vi "PC Streaming Host with slow.vi"() -> ()   [LabVIEW 2012]
uses:
  <vilib>/userdefined/High Color/nirio_resource_hc.ctl
  <vilib>/FPGAPlugInAG/PXI-7951R/niLvFpga_Open_PXI-7951R.vi
  <vilib>/rvi/interface/common/dynamic/niFpgaDynamicAddResources.vi
  <vilib>/Utility/error.llb/Error Cluster From Error Code.vi
  <vilib>/rvi/errors/niLvFpgaAdjustHostInterfaceError.vi
  <vilib>/FPGAPlugInAG/Dynamic/niLvFpga_Close_Dynamic.vi
  <vilib>/rvi/interface/nirviOpenFPGA/nirviOpenFPGA.xnode
  FPGA Bitfiles/ModuDAQ_FPGATarget_TopLevelFPGAw8ra_+uETqx0Rcow.lvbitx
  <vilib>/rvi/interface/nirviReadWriteControl/nirviReadWriteControl.xnode
  <vilib>/rvi/interface/nirviMethod/nirviMethod.xnode
  <vilib>/rvi/interface/nirviCloseFPGA/nirviCloseFPGA.xnode
  <vilib>/rvi/errors/niLvFpgaMergeErrorWithErrorCode.vi
  <vilib>/ptbypt/NI_PtbyPt.lvlib
  <vilib>/rvi/interface/Simulation/niFpgaSimulationCallBeginRW.vi
  RT_binary.vi
  NiFpgaLv.dll
  <vilib>/FPGAPlugInAG/Dynamic/niLvFpga_ReadFifo_Dynamic.vi
panel:
  out "created path":path
  out "File name":string
  out "Total Data Chunks to Write":dbl
  in  "Tab Control":T1(tab)
  in  "Write mode":bool
  out "directory exists - please wait":u8(slide)
  out "directory ok":bool
  in  "Write Enable":bool
  in  "File Path":path=path "D:/Users/reuterc/Desktop"
  out "File Writing Progress (%)":dbl(slide) scale=0.0..100.0
  in  "Slow Control On":bool
  in  "Fast Data On":bool
  in  "Number of Files to Write":u32=1
  in  "IP Address of NIST Time Server":string(combo)
  in  "VISA resource name":refnum<visa-resource-name>="COM5"
  in  "General Cluster":cluster{"Location":i16} {"Location" items=["Purdue", "NIKHEF", "Zurich", "???"]}
  in  "PXI address":T2 caption="RIO Device"
  in  "Channel Cluster":T3={"det_type"=[], "voltage"=[], "Serial numbers"=[], "Sources"=[], "Trigger level"=[4000, 4000, 4000, 4000, 4000, 4000, 4000, 4000], "Channel On/Off"=[], "Number of Channels"=8}
  in  "Testpulse Cluster":T4={"Master Pulser On/Off"=FALSE, "Testpulse Turnaround Time (samples)"=14, "Pulse Separation (samples)"=0, "Pulse duration (samples)"=0}
  out "Samples per Data Chunk":u32
  in  "DAQ Info Cluster":T5={"Data Chunks per File"=1000, "Samples per Waveform"=95, "Pretrigger Samples"=15, "circular buffer length (samples)"=1000, "Waveforms per Data Chunk"=5000} {"Waveforms per Data Chunk" format="%.2p"}
  out "Average Throughput":dbl(graph)
  out "Loop Time":u32
  out "Inst. Throughput":dbl format="%#_6p"
  out "Elements in FIFO":u32(graph)
  out "FIFO Overflow":bool
  out "Current Chunk":u32
  out "Current File":i32
  out "Waveform Graph":dynamicdata(graph)
  out "Channel number displayed":i16=-1
  in  "Arduino read rate (Hz)":dbl=1.0
  out "read buffer":string
  out "array 2":string[](array[string])
  out "Arduino read failed":bool
  out "Slow time":u64
  out "data":dbl[](array[numeric])
  in  "XON Character":u8=17 format="%.0x"
  in  "XOFF Character":u8=19 format="%.0x"
  out "Slow Cluster":T6={"Number of Slow Parameters"=0, "UTC format?"=TRUE, "Sensor Upper bounds"=[85, 1000000, 8000, 8000, 8000, 14000, 99, 33000], "Sensor Lower bounds"=[-40, 0, -8000, -8000, -8000, -14000, 0, -33000], "datanames"=[], "Descriptions"=[]}
  out "Number of Slow Parameters":i32
  out "FPGA Timestamp (s)":u64
  out "Temperature":dbl(graph)
  out "Pressure":dbl(graph)
  out "magnetic field y coordinate":dbl(graph)
  out "total magnetic field":dbl(graph)
  out "magnetic field z coordinate":dbl(graph)
  out "magnetic field x coordinate":dbl(graph)
  out "humidity":dbl(graph)
  out "XML String":string
  out "error out":errorcluster
  out "NIST Time":u64
  out "NIST Time Failed to Read":bool
  in  "Minutes to wait":u32=5 min=3
  out "UTC format":bool=TRUE
  out "Stopped":bool
  in  "stop 2":bool
  in  "stop":bool
  # "Write continuously"
  # "Write finite number of files"
  # "Program will stop when number of Files to Write is Complete OR if stop is pressed."
  # "TODO: Make this look like the \"detectors\" tab"
  # "Waveform/Data Chunk information"
  # "To compare directly on a scope: Horizontal scale: 200 ns/div Vertical scale: ~100 mV/div If 15 pretriggers, delay = 700 ns"
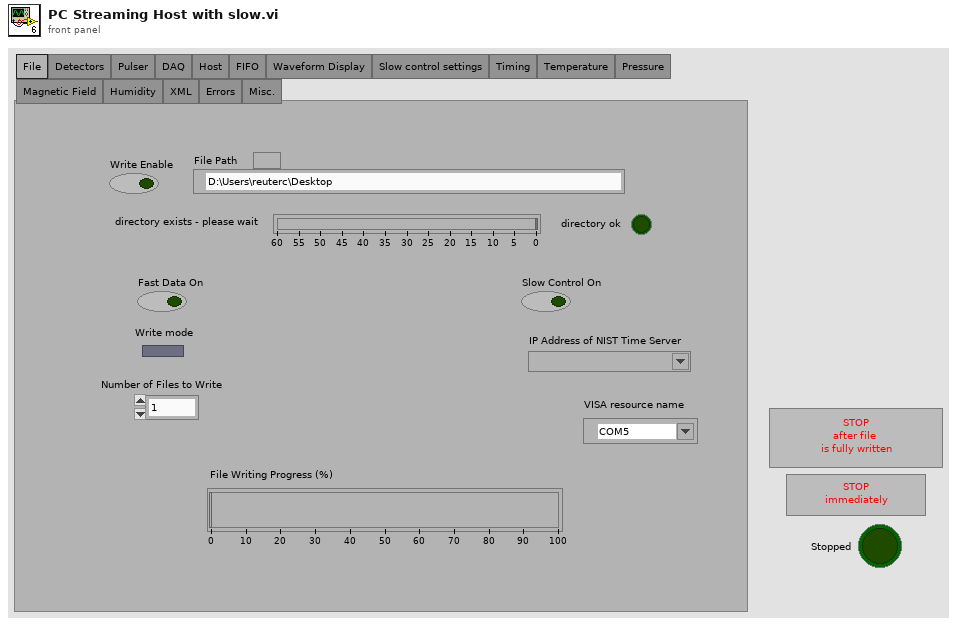
[diagram p1: front panel]
types:
  T1 = enum32{"File", "Detectors", "Pulser", "DAQ", "Host", "FIFO", "Waveform Display", "Slow control settings", "Timing", "Temperature", "Pressure", "Magnetic Field", "Humidity", "XML", "Errors", "Misc."}
  T2 = typedef "nirio_resource_hc.ctl" = tag
  T3 = cluster{"det_type":string[], "voltage":string[], "Serial numbers":string[], "Sources":string[], "Trigger level":i16[], "Channel On/Off":bool[], "Number of Channels":u8}
  T4 = cluster{"Master Pulser On/Off":bool, "Testpulse Turnaround Time (samples)":u32, "Pulse Separation (samples)":u32, "Pulse duration (samples)":u32}
  T5 = cluster{"Data Chunks per File":u32, "Samples per Waveform":u32, "Pretrigger Samples":u32, "circular buffer length (samples)":u32, "Waveforms per Data Chunk":u32}
  T6 = cluster{"Number of Slow Parameters":i32, "UTC format?":bool, "Sensor Upper bounds":i32[], "Sensor Lower bounds":i32[], "datanames":string[], "Descriptions":string[]}
  T7 = enum16{"open", "replace", "create", "open or create", "replace or create", "replace or create with confirmation"}
  T8 = enum16{"big-endian, network order", "native, host order", "little-endian"}
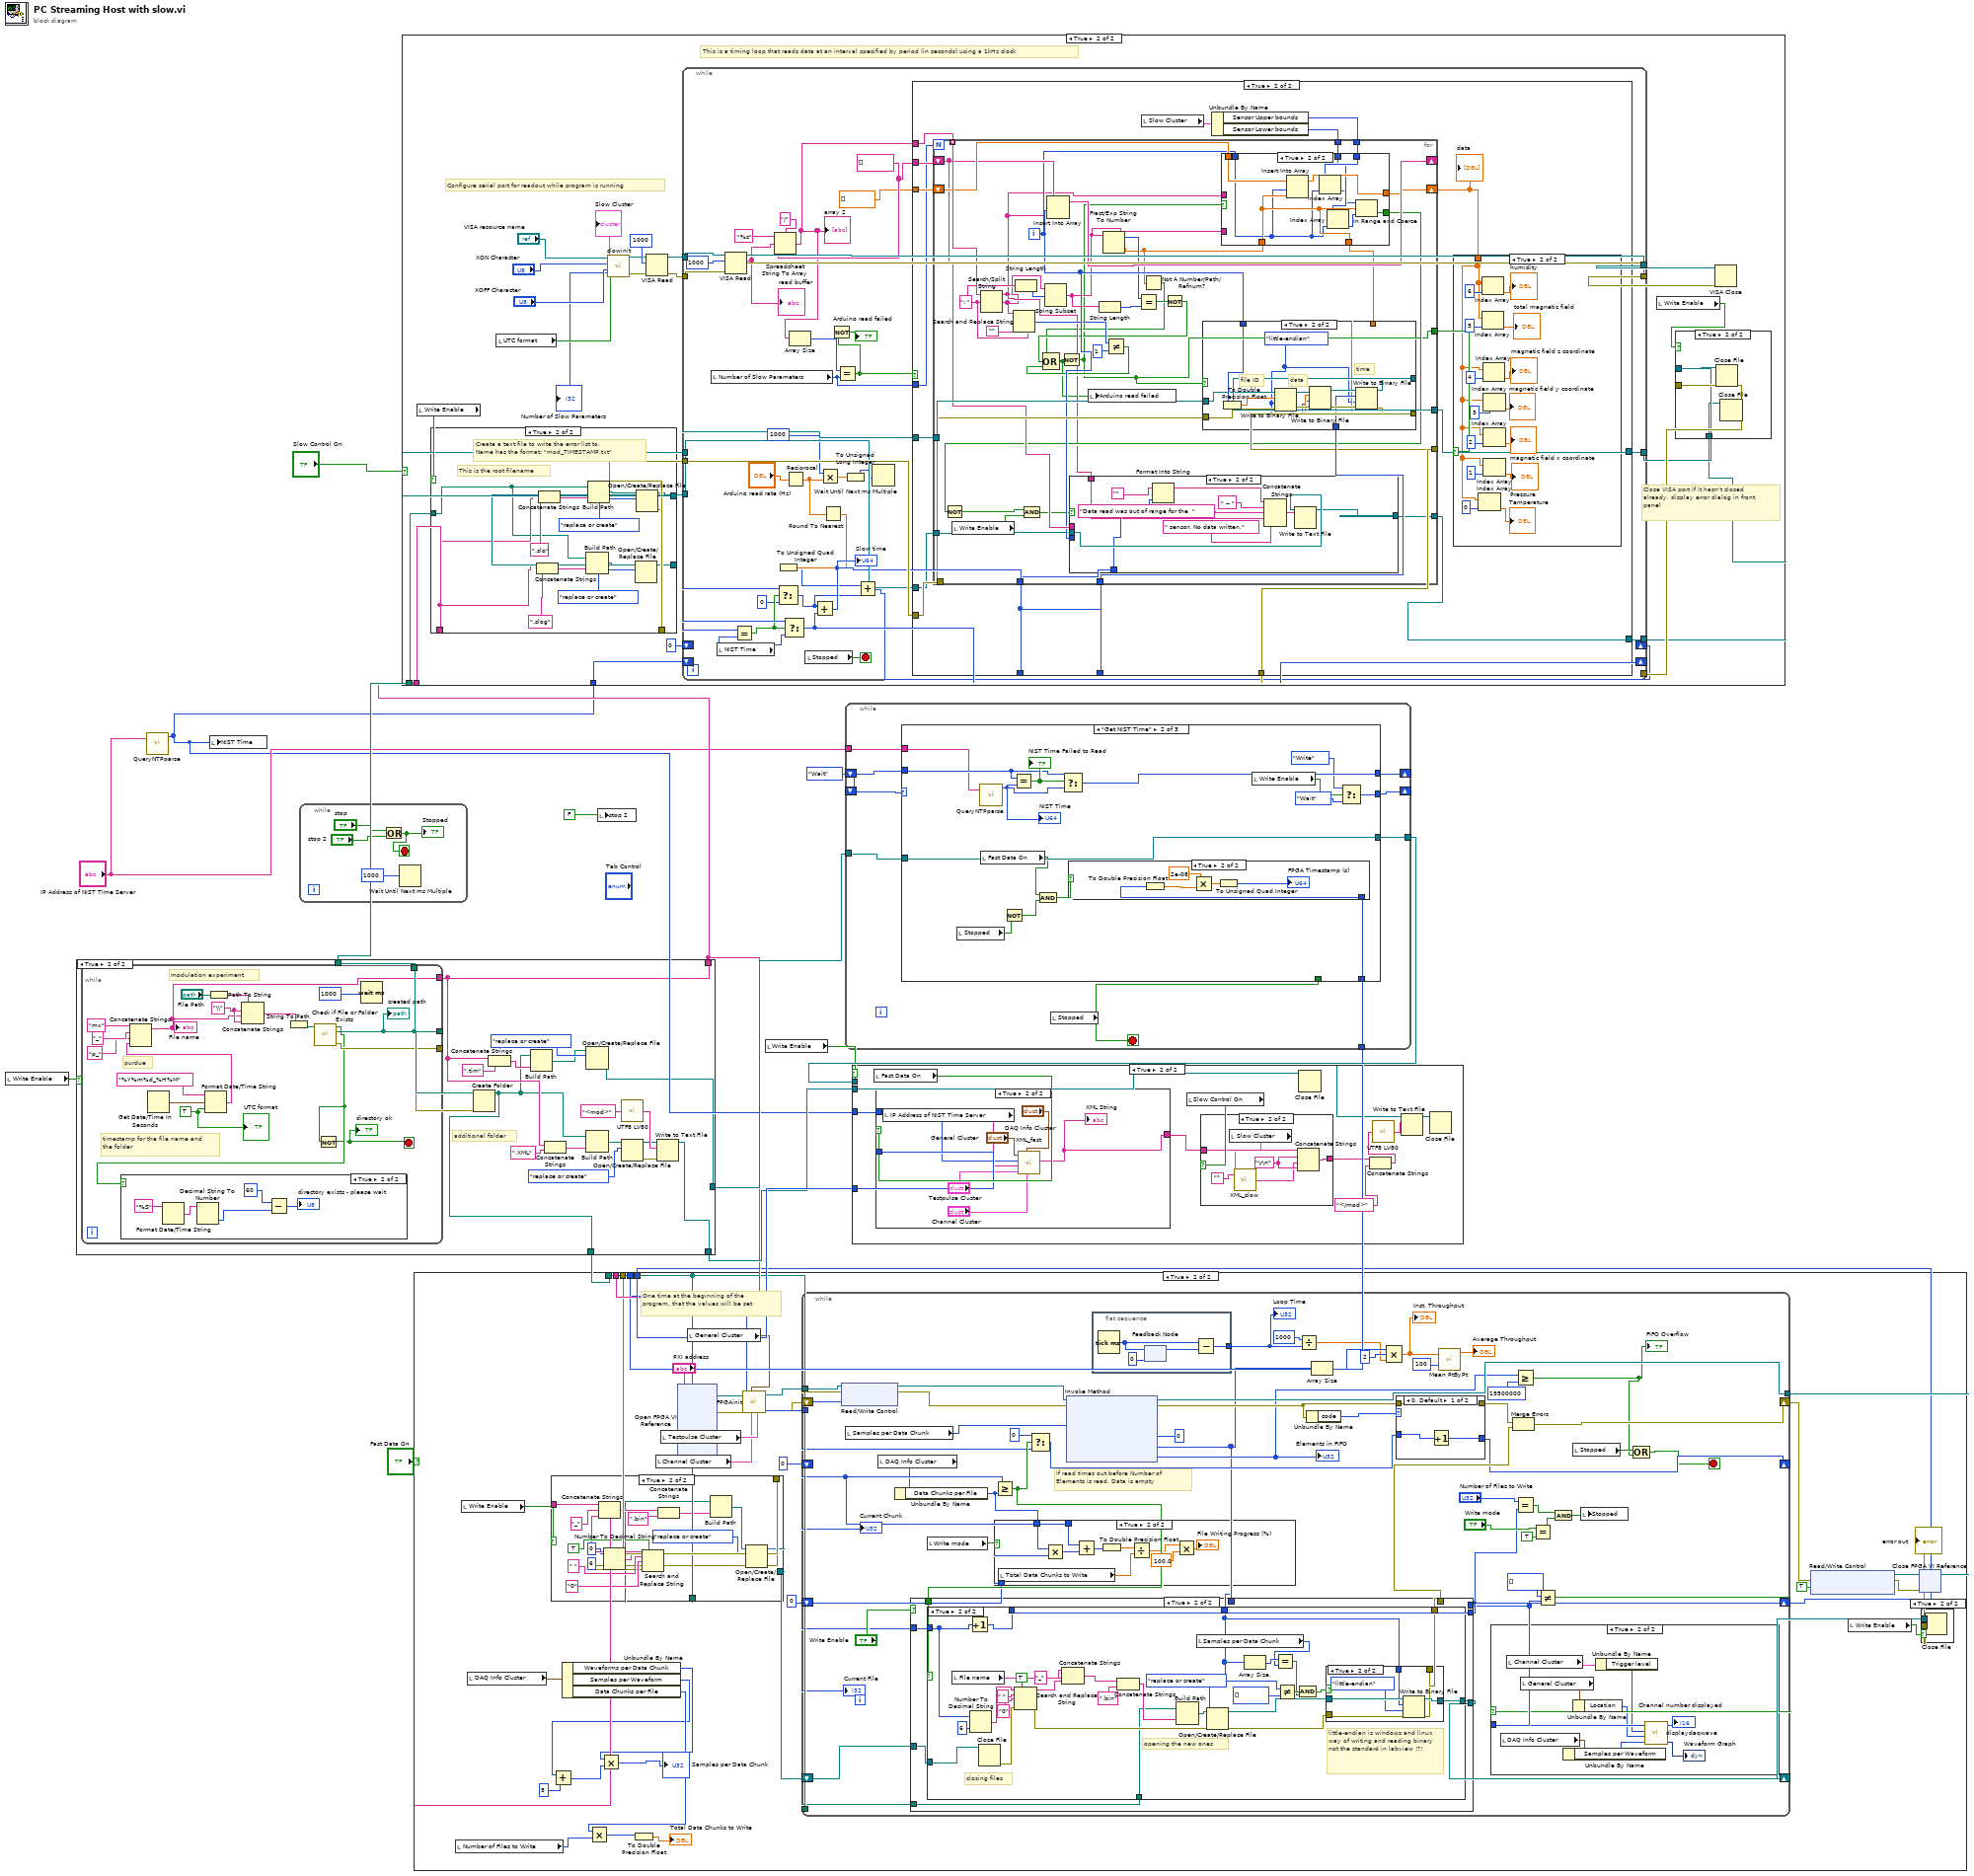
[diagram p0: block diagram]
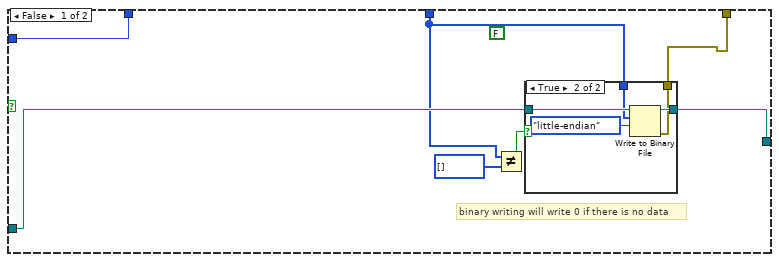
[diagram p7: hidden frame]
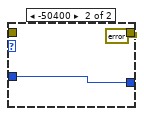
[diagram p10: hidden frame]
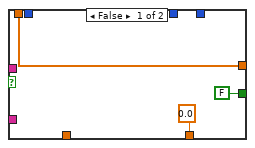
[diagram p15: hidden frame]
diagram:
  n1 = local read "Write Enable"() -> (w12:bool)
  n2 = case shown="True" w12 {
    tunnel: [_ w33] -> w14
    tunnel: [_ w28] -> w8
    tunnel: [_ w20] -> w6
    tunnel: [_ w18] -> w5
    tunnel: [_ w17] -> w3
    frame False {
    }
    frame True {
      # "additional folder"
      n3 = while {
        tunnel: [w46] -> w30
        tunnel: [w37] -> w31
        tunnel: [w37] -> w28
        tunnel: [w36] -> w18
        stop <- w43 stop-if-true
        w38 = "\\" ("string")
        w49 = TRUE ("UTC format")
        # "modulation experiment"
        # "purdue"
        # "timestamp for the file name and the folder"
        n4 = Get Date/Time In Seconds() -> (seconds since 1Jan1904=w50:timestamp)
        n5 = Format Date/Time String(time format string (%c)="%Y%m%d_%H%M", seconds (now)=w50, UTC format=w49) -> (date/time string=w39:string)
        n6 = Concatenate Strings("mx" ("string"), "_" ("string"), "p_" ("string"), w39) -> (w36:string)
        "File name" <- w36
        n7 = Path To String(path="File Path") -> (string=w52:string)
        n8 = Concatenate Strings(w52, w38, w36, w38) -> (w53:string)
        n9 = String To Path(string=w53) -> (path=w47:path)
        n10 = call <vilib>:"Check if File or Folder Exists.vi"("path"=w47) -> ("error out"=w46:errorcluster, "file or folder exists?"=w45:bool, "dup path"=w37:path)  [unwired: 8 in]
        "created path" <- w37
        n11 = case shown="True" w45 {
          frame False {
          }
          frame True {
            n12 = Format Date/Time String(time format string (%c)="%S") -> (date/time string=w57:string)  [unwired: 2 in]
            n13 = Decimal String To Number(string=w57) -> (number=w55:i32)  [unwired: 2 in, 1 out]
            n14 = Subtract(x=60, y=w55) -> (x-y=→"directory exists - please wait":i32)
          }
        }
        n15 = Not(x=w45) -> (.not. x?=w43:bool)
        "directory ok" <- w43
        n16 = Wait (ms)(milliseconds to wait=1000) -> ()  [unwired: 1 out]
        "UTC format" <- w49
      }
      n17 = Create Folder(path (use dialog)=w31, error in=w30) -> (created path=w17:path)  [unwired: 1 in, 2 out]
      n18 = Concatenate Strings(w18, ".tim" ("string")) -> (w32:string)
      n19 = Build Path(base path=w17, name or relative path=w32) -> (appended path=w29:path)
      n20 = Concatenate Strings(w18, ".XML" ("substring (\"\")")) -> (w24:string)
      n21 = Open/Create/Replace File(file path (use dialog)=w29, operation (0:open)=T7."replace or create") -> (refnum out=w33:refnum<file>)  [unwired: 4 in, 2 out]
      n22 = Build Path(base path=w17, name or relative path=w24) -> (appended path=w23:path)
      n23 = call "UTF8 LV80.vi"("text"="<mod>") -> ("utf-8 text out"=w27:string)
      n24 = Open/Create/Replace File(file path (use dialog)=w23, operation (0:open)=T7."replace or create") -> (refnum out=w26:refnum<file>, error out=w25:errorcluster)  [unwired: 4 in, 1 out]
      n25 = Write to Text File(file (use dialog)=w26, text=w27, error in=w25) -> (refnum out=w20:refnum<file>)  [unwired: 1 in, 2 out]
    }
  }
  n26 = call "QueryNTPparse.vi"("IP Address of NIST Server"="IP Address of NIST Time Server") -> ("NTP Time"=w1:u64)  [unwired: 1 in, 2 out]
  n27 = local write "NIST Time"(w1) -> ()
  n28 = while {
    stop <- w59 stop-if-true
    n29 = Or(x="stop", y="stop 2") -> (x .or. y?=w59:bool)
    "Stopped" <- w59
    n30 = Wait Until Next ms Multiple(millisecond multiple=u32 1000 ("y")) -> ()  [unwired: 1 out]
  }
  n31 = case shown="True" "Slow Control On" {
    tunnel: w8 -> [_ w79]
    tunnel: w1 -> [_ w77]
    tunnel: w5 -> [_ w76]
    frame False {
    }
    frame True {
      # "This is a timing loop that reads data at an interval specified by period (in seconds) using a 1kHz clock"
      # "Configure serial port for readout while program is running"
      # "Close VISA port if it hasn't closed already, display error dialog in front panel"
      n32 = local read "Write Enable"() -> (w86:bool)
      n33 = case shown="True" w86 {
        tunnel: [_ w250] -> w83
        tunnel: [_ w247] -> w81
        tunnel: w79 -> [_ w240]
        tunnel: w76 -> [_ w242]
        tunnel: [_ w241] -> w72
        frame False {
        }
        frame True {
          # "This is the root filename"
          # "Create a text file to write the error list to.  \nName has the format: \"mod_TIMESTAMP.txt\""
          n34 = Concatenate Strings(w242, ".slog") -> (w243:string)
          n35 = Concatenate Strings(w242, ".slo") -> (w248:string)
          n36 = Build Path(base path=w240, name or relative path=w243) -> (appended path=w244:path)
          n37 = Build Path(base path=w240, name or relative path=w248) -> (appended path=w249:path)
          n38 = Open/Create/Replace File(file path (use dialog)=w244, operation (0:open)=T7."replace or create") -> (refnum out=w241:refnum<file>)  [unwired: 4 in, 2 out]
          n39 = Open/Create/Replace File(file path (use dialog)=w249, operation (0:open)=T7."replace or create") -> (refnum out=w250:refnum<file>, error out=w247:errorcluster)  [unwired: 4 in, 1 out]
        }
      }
      n40 = local read "UTC format"() -> (w67:bool)
      n41 = call "slowinit.vi"("UTC format"=w67, "XOFF Character"="XOFF Character", "XON Character"="XON Character", "VISA resource name"="VISA resource name") -> ("error IO"=w64:errorcluster, "VISA resource name out"=w66:refnum<visa-resource-name>, "Number of Slow Parameters"=→"Number of Slow Parameters":i32, "Slow Cluster"=→"Slow Cluster":T6)  [unwired: 4 in]
      n42 = VISA Read(VISA resource name=w66, byte count=u32 1000, error in (no error)=w64) -> (VISA resource name out=w75:refnum<visa-resource-name>, error out=w74:errorcluster)  [unwired: 2 out]
      n43 = while {
        tunnel: w75 -> [w124]
        tunnel: w74 -> [w123]
        tunnel: [w122] -> w85
        tunnel: [w121] -> w84
        shift-right: [w111] -> _
        shift-left: w77 -> [w115]
        shift-right: [w96] -> _
        shift-left: 0 -> [w113]
        tunnel: w81 -> [w109]
        tunnel: [w108] -> w80
        tunnel: w83 -> [w117]
        tunnel: [w107] -> w78
        tunnel: w72 -> [w104]
        tunnel: [w102] -> w71
        stop <- w110 stop-if-true
        w101 = string[] [] ("array type (2D Dbl)")
        n44 = local read "Number of Slow Parameters"() -> (w88:i32)
        n45 = local read "NIST Time"() -> (w116:u64)
        n46 = VISA Read(VISA resource name=w124, byte count=u32 1000, error in (no error)=w123) -> (VISA resource name out=w122:refnum<visa-resource-name>, read buffer=w120:string, error out=w121:errorcluster)  [unwired: 1 out]
        "read buffer" <- w120
        n47 = Equal?(x=w115, y=w116) -> (x = y?=w114:bool)
        n48 = Spreadsheet String To Array(delimiter (Tab)="/", format string="%s", spreadsheet string=w120, array type (2D Dbl)=w101) -> (array=w90:string[])
        "array 2" <- w90
        n49 = Select(t=w113, s=w114, f=0) -> (s? t:f=w97:u64)
        n50 = Select(t=w115, s=w114, f=w116) -> (s? t:f=w111:u64)
        n51 = Reciprocal(x="Arduino read rate (Hz)") -> (1/x=w93:dbl)
        n52 = Array Size(array=w90) -> (size(s)=w89:i32)
        n53 = local read "Stopped"() -> (w110:bool)
        n54 = Add(x=w97, y=w111) -> (x+y=w103:u64)
        "Slow time" <- w103
        n55 = Multiply(x=u32 1000 ("millisecond multiple"), y=w93) -> (x*y=w95:dbl)
        n56 = Round To Nearest(number=w93) -> (nearest integer value=w92:dbl)
        n57 = To Unsigned Quad Integer(1:w92) -> (0:w91:u64)
        n58 = Equal?(x=w89, y=w88) -> (x = y?=w106:bool)
        n59 = Not(x=w106) -> (.not. x?=→"Arduino read failed":bool)
        n60 = To Unsigned Long Integer(number=w95) -> (unsigned 32bit integer=w94:u32)
        n61 = Add(x=w91, y=w97) -> (x+y=w96:u64)
        n62 = Wait Until Next ms Multiple(millisecond multiple=w94) -> ()  [unwired: 1 out]
        n63 = case shown="True" w106 {
          tunnel: w90 -> [_ w145]
          tunnel: w101 -> [_ w144]
          tunnel: w117 -> [w127 w143]
          tunnel: w103 -> [_ w142]
          tunnel: w109 -> [w128 w141]
          tunnel: [w128 w140] -> w108
          tunnel: [w127 w139] -> w107
          tunnel: w104 -> [w126 w137]
          tunnel: w103 -> [_ w136]
          tunnel: [w126 w135] -> w102
          tunnel: dbl[] [] ("array type (2D Dbl)") -> [_ w133]
          tunnel: w88 -> [_ w129]
          frame False {
          }
          frame True {
            n64 = local read "Slow Cluster"() -> (w132:T6)
            n65 = Unbundle By Name(w132) -> ("Sensor Upper bounds"=w131:i32[], "Sensor Lower bounds"=w130:i32[])
            n66 = for {
              N: w129 -> [_]
              tunnel: w145 -> [w198] mode=indexing
              shift-right: [w197] -> _
              shift-left: w144 -> [w188]
              shift-right: [w195] -> w138
              shift-left: w133 -> [w196]
              tunnel: w143 -> [w194]
              tunnel: [w193] -> w139
              tunnel: w142 -> [w192]
              tunnel: w141 -> [w191]
              tunnel: [w190] -> w140
              tunnel: w137 -> [w186]
              tunnel: w136 -> [w185]
              tunnel: [w184] -> w135
              tunnel: [w163] -> w134
              tunnel: w131 -> [w162]
              tunnel: w130 -> [w161]
              i -> [w187]
              w173 = ": " ("search string/char (-)")
              n67 = local read "Write Enable"() -> (w174:bool)
              n68 = Search/Split String(string=w198, search string/char (-)=w173) -> (substring before match=w171:string, match + rest of string=w169:string)  [unwired: 1 in, 1 out]
              n69 = Search and Replace String(input string=w169, search string=w173, replace string="") -> (number of replacements=w178:i32)  [unwired: 5 in, 3 out]
              n70 = String Length(string=w173) -> (length=w172:i32)
              n71 = String Subset(string=w169, offset (0)=w172) -> (substring=w170:string)  [unwired: 1 in]
              n72 = Insert Into Array(array=w188, index=w187, new element=w171) -> (w197:string[])
              n73 = String Length(string=w170) -> (length=w181:i32)
              n74 = Fract/Exp String To Number(string=w170) -> (offset past number=w182:i32, number=w166:dbl)  [unwired: 3 in]
              n75 = Not Equal?(x=w178, y=1) -> (x != y?=w176:bool)
              n76 = Equal?(x=w182, y=w181) -> (x = y?=w180:bool)
              n77 = Not A Number/Path/Refnum?(number/path/refnum=w166) -> (NaN/Path/Refnum?=w165:bool)
              n78 = Not(x=w180) -> (.not. x?=w167:bool)
              n79 = Compound Arithmetic op=OR(w165, w167, w176) -> (w168:bool)
              n80 = Not(x=w168) -> (.not. x?=w163:bool)
              n81 = local write "Arduino read failed"(w168) -> ()
              n82 = case shown="True" w163 {
                tunnel: w196 -> [w199 w210]
                tunnel: [w199 w208] -> w195
                tunnel: w171 -> [_ _]
                tunnel: [0.0 w207] -> w189
                tunnel: w187 -> [_ w206]
                tunnel: [FALSE w209] -> w183
                tunnel: w170 -> [_ _]
                tunnel: w166 -> [_ w207]
                tunnel: w162 -> [_ w205]
                tunnel: w161 -> [_ w204]
                frame False {
                }
                frame True {
                  n83 = Insert Into Array(array=w210, index=w206, new element=w207) -> (w208:dbl[])
                  n84 = Index Array(array=w205, index=w206) -> (element=w203:i32)
                  n85 = Index Array(array=w204, index=w206) -> (element=w202:i32)
                  n86 = In Range and Coerce(upper limit=w203, x=w207, lower limit=w202) -> (In Range?=w209:bool)  [unwired: 1 out]
                }
              }
              n87 = Not(x=w183) -> (.not. x?=w175:bool)
              n88 = And(x=w175, y=w174) -> (x .and. y?=w164:bool)
              n89 = case shown="True" w164 {
                tunnel: w188 -> [_ _]
                tunnel: w187 -> [_ _]
                tunnel: w186 -> [w211 w219]
                tunnel: w185 -> [_ w217]
                tunnel: [w211 w215] -> w184
                tunnel: w171 -> [_ w212]
                frame False {
                }
                frame True {
                  n90 = Format Into String(initial string="", w217) -> (resulting string=w216:string)  [unwired: 2 in, 1 out]
                  n91 = Concatenate Strings(w216, " -- " ("format string"), "Data read was out of range for the  " ("format string"), w212, " sensor. No data written." ("format string")) -> (w213:string)
                  n92 = Write to Text File(file (use dialog)=w219, text=w213) -> (refnum out=w215:refnum<file>)  [unwired: 2 in, 2 out]
                }
              }
              n93 = case shown="True" w163 {
                tunnel: [w223 w230] -> w193
                tunnel: w194 -> [w223 w233]
                tunnel: w187 -> [_ w234]
                tunnel: w192 -> [_ w227]
                tunnel: w191 -> [w222 w236]
                tunnel: [w222 w228] -> w190
                tunnel: w189 -> [_ w226]
                frame False {
                }
                frame True {
                  w224 = T8."little-endian" ("byte order (0:big-endian, network order)")
                  # "time"
                  # "data"
                  # "file ID"
                  n94 = To Double Precision Float(number=w234) -> (double precision float=w225:dbl)
                  n95 = Write to Binary File(file (use dialog)=w233, data=w225, error in=w236, 9:w224) -> (refnum out=w232:refnum<file>, error out=w235:errorcluster)  [unwired: 2 in, 1 out]
                  n96 = Write to Binary File(file (use dialog)=w232, data=w226, error in=w235, 9:w224) -> (refnum out=w231:refnum<file>, error out=w229:errorcluster)  [unwired: 2 in, 1 out]
                  n97 = Write to Binary File(file (use dialog)=w231, data=w227, error in=w229, 9:w224) -> (refnum out=w230:refnum<file>, error out=w228:errorcluster)  [unwired: 2 in, 1 out]
                }
              }
            }
            "data" <- w138
            n98 = case shown="True" w134 {
              tunnel: w138 -> [_ w153]
              frame False {
              }
              frame True {
                n99 = Index Array(array=w153, index=0) -> (element=→"Temperature":dbl)
                n100 = Index Array(array=w153, index=6) -> (element=→"humidity":dbl)
                n101 = Index Array(array=w153, index=5) -> (element=→"total magnetic field":dbl)
                n102 = Index Array(array=w153, index=4) -> (element=→"magnetic field z coordinate":dbl)
                n103 = Index Array(array=w153, index=3) -> (element=→"magnetic field y coordinate":dbl)
                n104 = Index Array(array=w153, index=2) -> (element=→"magnetic field x coordinate":dbl)
                n105 = Index Array(array=w153, index=1) -> (element=→"Pressure":dbl)
              }
            }
          }
        }
      }
      n106 = local read "Write Enable"() -> (w87:bool)
      n107 = case shown="True" w87 {
        tunnel: w78 -> [_ w239]
        tunnel: w80 -> [_ w238]
        tunnel: w71 -> [_ w237]
        frame False {
        }
        frame True {
          n108 = Close File(refnum=w239, error in=w238) -> ()  [unwired: 2 out]
          n109 = Close File(refnum=w237) -> ()  [unwired: 1 in, 2 out]
        }
      }
      n110 = VISA Close(VISA resource name=w85, error in (no error)=w84) -> ()  [unwired: 1 out]
    }
  }
  n111 = case shown="True" "Fast Data On" {
    tunnel: [_ w287] -> _
    tunnel: [_ w274] -> w7
    tunnel: w5 -> [_ w273]
    tunnel: w3 -> [_ w272]
    tunnel: [_ w271] -> w2
    frame False {
    }
    frame True {
      # "One time at the beginning of the program, that the values will be set"
      n112 = local read "Number of Files to Write"() -> (w257:u32)
      n113 = local read "Write Enable"() -> (w286:bool)
      n114 = local read "DAQ Info Cluster"() -> (w269:T5)
      n115 = case shown="True" w286 {
        tunnel: [_ w432] -> w287
        tunnel: [_ w440] -> w285
        tunnel: w273 -> [_ w431]
        tunnel: w272 -> [_ w430]
        frame False {
        }
        frame True {
          n116 = Number To Decimal String(number=0, width (-)=i16 6) -> (decimal integer string=w447:string)
          n117 = Search and Replace String(replace all?=TRUE ("replace all? (F)"), input string=w447, search string=" ", replace string="0" ("replace string (\"\")")) -> (result string=w437:string, error out=w442:errorcluster)  [unwired: 4 in, 2 out]
          n118 = Concatenate Strings(w431, "_" ("string"), w437) -> (w435:string)
          n119 = Concatenate Strings(w435, ".bin" ("substring (\"\")")) -> (w439:string)
          n120 = Build Path(base path=w430, name or relative path=w439) -> (appended path=w443:path)
          n121 = Open/Create/Replace File(file path (use dialog)=w443, error in=w442, operation (0:open)=T7."replace or create") -> (refnum out=w440:refnum<file>, error out=w432:errorcluster)  [unwired: 3 in, 1 out]
        }
      }
      n122 = Unbundle By Name(w269) -> ("Waveforms per Data Chunk"=w254:u32, "Samples per Waveform"=w255:u32, "Data Chunks per File"=w256:u32)
      n123 = Add(x=w255, y=u32 5) -> (x+y=w259:u32)
      n124 = Multiply(x=w256, y=w257) -> (x*y=w261:u32)
      n125 = Multiply(x=w254, y=w259) -> (x*y=→"Samples per Data Chunk":u32)
      n126 = To Double Precision Float(number=w261) -> (double precision float=→"Total Data Chunks to Write":dbl)
      n127 = local read "Channel Cluster"() -> (w262:T3)
      n128 = local read "Testpulse Cluster"() -> (w264:T4)
      n129 = xnode "Open FPGA VI Reference"("resource name"="PXI address") -> ("FPGA VI Reference Out"=w268:refnum<k20>, "error out"=w267:errorcluster)  [unwired: 1 in]
      n130 = local read "General Cluster"() -> (w263:cluster{"Location":i16})
      n131 = call "FPGAinit.vi"("Testpulse Cluster"=w264, "Channel Cluster"=w262, "General Cluster"=w263, "error in"=w267, "FPGA VI Reference In"=w268) -> ("error out"=w265:errorcluster, "FPGA VI Reference Out"=w266:refnum<k20>)  [unwired: 5 in]
      n132 = while {
        shift-right: [w323] -> w277
        shift-left: w265 -> [w311]
        shift-right: [w319] -> _
        shift-left: u32 0 -> [w316]
        shift-right: [w300] -> w274
        shift-left: 0 ("number") -> [w304]
        shift-right: [w320] -> w281
        shift-left: w285 -> [w321]
        tunnel: [w339] -> w278
        tunnel: w272 -> [w312]
        tunnel: [w308] -> w271
        tunnel: w266 -> [w291]
        stop <- w305 stop-if-true
        # "If read times out before Number of Elements is read, Data is empty"
        n133 = xnode "Read/Write Control"("FPGA VI Reference In"=w291, "error in"=w311) -> ("FPGA VI Reference Out"=w310:refnum<k20>, "error out"=w309:errorcluster, "Timestamp"=w308:u64)
        n134 = local read "Samples per Data Chunk"() -> (w290:u32)
        n135 = local read "DAQ Info Cluster"() -> (w293:T5)
        n136 = Unbundle By Name(w293) -> ("Data Chunks per File"=w292:u32)
        n137 = local read "Write mode"() -> (w313:bool)
        n138 = Greater Or Equal?(x=w316, y=w292) -> (x >= y?=w325:bool)
        n139 = case shown="True" w313 {
          tunnel: w304 -> [_ w358]
          tunnel: w316 -> [_ w356]
          tunnel: w292 -> [_ w349]
          frame False {
          }
          frame True {
            n140 = local read "Total Data Chunks to Write"() -> (w353:dbl)
            n141 = Multiply(x=w349, y=w358) -> (x*y=w357:u32)
            n142 = Add(x=w356, y=w357) -> (x+y=w355:u32)
            n143 = To Double Precision Float(number=w355) -> (double precision float=w354:dbl)
            n144 = Divide(x=w354, y=w353) -> (x/y=w351:dbl)
            n145 = Multiply(x=w351, y=100.0) -> (x*y=→"File Writing Progress (%)":dbl)
          }
        }
        n146 = Select(t=u32 0, s=w325, f=w316) -> (s? t:f=w326:u32)
        n147 = xnode "Invoke Method"("FPGA VI Reference In"=w310, "error in"=w309, "Number of Elements"=w290, "Timeout (ms)"=0) -> ("FPGA VI Reference Out"=w339:refnum<k20>, "error out"=w336:errorcluster, "Data"=w314:i16[], "Elements Remaining"=w315:u32)
        "Elements in FIFO" <- w315
        n148 = case shown="True" "Write Enable" {
          tunnel: w314 -> [w364 w369]
          tunnel: [w364 _] -> w296
          tunnel: w325 -> [_ w373]
          tunnel: [_ w372] -> w322
          tunnel: [w365 w371] -> w320
          tunnel: w321 -> [w365 w370]
          tunnel: w312 -> [_ w368]
          tunnel: w304 -> [w363 w367]
          tunnel: [w363 w366] -> w300
          frame False {
          }
          frame True {
            n149 = case shown="True" w373 {
              tunnel: w369 -> [w376 w395]
              tunnel: [w375 w397] -> w372
              tunnel: w370 -> [w380 w410]
              tunnel: [w379 w403] -> w371
              tunnel: w368 -> [_ w390]
              tunnel: w367 -> [w374 w389]
              tunnel: [w374 w388] -> w366
              frame False {
                (unwired) FALSE
                # "binary writing will write 0 if there is no data"
                n150 = Not Equal?(x=w376, y=i16[] []) -> (x != y?=w377:bool)
                n151 = case shown="True" w377 {
                  tunnel: w380 -> [w381 w386]
                  tunnel: [w381 w385] -> w379
                  tunnel: [_ w384] -> w375
                  tunnel: w376 -> [_ w382]
                  frame False {
                  }
                  frame True {
                    n152 = Write to Binary File(file (use dialog)=w386, data=w382, 9:T8."little-endian" ("byte order (0:big-endian, network order)")) -> (refnum out=w385:refnum<file>, error out=w384:errorcluster)  [unwired: 3 in, 1 out]
                  }
                }
              }
              frame True {
                # "opening the new ones"
                # "closing files"
                # "little-endian is windows and linux way of writing and reading binary not the standard in labview !?!"
                n153 = local read "File name"() -> (w391:string)
                n154 = Increment(x=w389) -> (x+1=w388:i32)
                n155 = Number To Decimal String(number=w389, width (-)=i16 6) -> (decimal integer string=w412:string)
                n156 = Close File(refnum=w410) -> (error out=w409:errorcluster)  [unwired: 1 in, 1 out]
                n157 = Search and Replace String(replace all?=TRUE ("replace all? (F)"), input string=w412, search string=" ", replace string="0" ("replace string (\"\")"), error in=w409) -> (result string=w402:string, error out=w408:errorcluster)  [unwired: 3 in, 2 out]
                n158 = Concatenate Strings(w391, "_" ("string"), w402) -> (w398:string)
                n159 = Concatenate Strings(w398, ".bin" ("substring (\"\")")) -> (w400:string)
                n160 = Build Path(base path=w390, name or relative path=w400) -> (appended path=w407:path)
                n161 = local read "Samples per Data Chunk"() -> (w387:u32)
                n162 = Open/Create/Replace File(file path (use dialog)=w407, error in=w408, operation (0:open)=T7."replace or create") -> (refnum out=w404:refnum<file>, error out=w405:errorcluster)  [unwired: 3 in, 1 out]
                n163 = Array Size(array=w395) -> (size(s)=w394:i32)
                n164 = Equal?(x=w394, y=w387) -> (x = y?=w393:bool)
                n165 = Not Equal?(x=w395, y=i16[] []) -> (x != y?=w396:bool)
                n166 = And(x=w396, y=w393) -> (x .and. y?=w392:bool)
                n167 = case shown="True" w392 {
                  tunnel: w405 -> [w417 w424]
                  tunnel: w404 -> [w418 w423]
                  tunnel: [w418 w422] -> w403
                  tunnel: [w417 w421] -> w397
                  tunnel: w395 -> [_ w420]
                  frame False {
                  }
                  frame True {
                    n168 = Write to Binary File(file (use dialog)=w423, data=w420, error in=w424, 9:T8."little-endian" ("byte order (0:big-endian, network order)")) -> (refnum out=w422:refnum<file>, error out=w421:errorcluster)  [unwired: 2 in, 1 out]
                  }
                }
              }
            }
          }
        }
        n169 = flat-sequence {
          tunnel: [w362] -> w330
          frame #0 {
            n170 = Tick Count (ms)() -> (millisecond timer value=w361:u32)
            n171 = feedback #1(u32 0 ("millisecond timer value")) -> (w360:u32)
            n172 = feedback-in #1(w361) -> ()
            n173 = Subtract(x=w361, y=w360) -> (x-y=w362:u32)
          }
        }
        n174 = Divide(x=u32 1000, y=w330) -> (x/y=w332:dbl)
        n175 = Unbundle By Name(w336) -> ("code"=w337:i32)
        n176 = Array Size(array=w314) -> (size(s)=w335:i32)
        n177 = Compound Arithmetic op=MULTIPLY(w335, 2 ("y"), w332) -> (w329:dbl)
        "Inst. Throughput" <- w329
        n178 = case shown="0, Default" w337 {
          tunnel: [w427 errorcluster {"status"=FALSE, "code"=0, "source"=""} ("error constant")] -> w324
          tunnel: w336 -> [w427 _]
          tunnel: w326 -> [w426 w428]
          tunnel: [w425 w428] -> w319
          frame 0, Default {
            n179 = Increment(x=w426) -> (x+1=w425:u32)
          }
          frame -50400 {
          }
        }
        n180 = call <vilib>:"Mean PtByPt.vi"("x"=w329, "sample length"=100) -> ("mean"=→"Average Throughput":dbl)  [unwired: 2 in, 1 out]
        n181 = Merge Errors(w324, w322) -> (w323:errorcluster)
        n182 = Greater Or Equal?(x=w315, y=u32 19500000) -> (x >= y?=w306:bool)
        "FIFO Overflow" <- w306
        n183 = Equal?(x="Number of Files to Write", y=w300) -> (x = y?=w299:bool)
        n184 = Equal?(x="Write mode", y=TRUE) -> (x = y?=w298:bool)
        n185 = Not Equal?(x=i16[] [], y=w296) -> (x != y?=w294:bool)
        n186 = case shown="True" w294 {
          tunnel: w296 -> [_ w348]
          frame False {
          }
          frame True {
            n187 = local read "DAQ Info Cluster"() -> (w341:T5)
            n188 = local read "Channel Cluster"() -> (w345:T3)
            n189 = local read "General Cluster"() -> (w343:cluster{"Location":i16})
            n190 = Unbundle By Name(w341) -> ("Samples per Waveform"=w340:u32)
            n191 = Unbundle By Name(w343) -> ("Location"=w342:i16)
            n192 = Unbundle By Name(w345) -> ("Trigger level"=w344:i16[])
            n193 = call "displaydaqwave.vi"("Samples per Waveform"=w340, "Location"=w342, "Trigger level"=w344, "Waveform from DAQ"=w348) -> ("Waveform Graph"=→"Waveform Graph":dynamicdata, "Channel number displayed"=→"Channel number displayed":i16)  [unwired: 6 in]
          }
        }
        n194 = And(x=w299, y=w298) -> (x .and. y?=w297:bool)
        n195 = local read "Stopped"() -> (w307:bool)
        n196 = local write "Stopped"(w297) -> ()
        n197 = Compound Arithmetic op=OR(w307, w306) -> (w305:bool)
        "Loop Time" <- w330
        "Current Chunk" <- w316
        "Current File" <- w304
      }
      n198 = xnode "Read/Write Control"("FPGA VI Reference In"=w278, "error in"=w277, "Stop FPGA and exit"=TRUE) -> ("FPGA VI Reference Out"=w270:refnum<k20>, "error out"=w280:errorcluster)
      n199 = local read "Write Enable"() -> (w283:bool)
      n200 = xnode "Close FPGA VI Reference"("FPGA VI Reference In"=w270, "error in"=w280) -> ("error out"=w284:errorcluster)
      "error out" <- w284
      n201 = case shown="True" w283 {
        tunnel: w284 -> [_ w288]
        tunnel: w281 -> [_ w289]
        frame False {
        }
        frame True {
          n202 = Close File(refnum=w289, error in=w288) -> ()  [unwired: 2 out]
        }
      }
    }
  }
  n203 = local write "stop 2"(FALSE ("stop 2")) -> ()
  n204 = local read "Write Enable"() -> (w11:bool)
  n205 = while {
    shift-right: [w455] -> _
    shift-left: enum16{"Wait", "Get NIST Time", "Write"}."Wait" -> [w456]
    shift-right: [w454] -> _
    shift-left: _ -> [w453]
    tunnel: w14 -> [w452]
    tunnel: [w451] -> w13
    tunnel: "IP Address of NIST Time Server" -> [w450]
    tunnel: w2 -> [w448]
    stop <- w449 stop-if-true
    n206 = local read "Stopped"() -> (w449:bool)
    n207 = case shown="\"Get NIST Time\"" w456 {
      tunnel: [w461 w477 enum16{"Wait", "Get NIST Time", "Write"}."Wait"] -> w455
      tunnel: [w460 w485 w495] -> w454
      tunnel: w453 -> [w460 w482 w495]
      tunnel: w452 -> [w459 w481 w501]
      tunnel: [w459 w481 w500] -> w451
      tunnel: w449 -> [w458 _ _]
      tunnel: w450 -> [_ w476 _]
      tunnel: w448 -> [_ w471 _]
      frame "Wait", Default {
        n208 = while {
          tunnel: [enum16{"Wait", "Get NIST Time", "Write"}."Get NIST Time"] -> w461
          tunnel: w458 -> [_]
          tunnel: "Minutes to wait" -> [w463]
          i -> [w466]
          stop <- w467 stop-if-true
          n209 = Multiply(x=60, y=w463) -> (x*y=w462:u32)
          n210 = Greater Or Equal?(x=w466, y=w462) -> (x >= y?=w468:bool)
          n211 = local read "Stopped"() -> (w465:bool)
          n212 = Or(x=w468, y=w465) -> (x .or. y?=w467:bool)
          n213 = Wait Until Next ms Multiple(millisecond multiple=u32 1000 ("y")) -> ()  [unwired: 1 out]
        }
      }
      frame "Get NIST Time" {
        n214 = local read "Stopped"() -> (w472:bool)
        n215 = call "QueryNTPparse.vi"("IP Address of NIST Server"=w476) -> ("NTP Time"=w484:u64)  [unwired: 1 in, 2 out]
        "NIST Time" <- w484
        n216 = local read "Fast Data On"() -> (w475:bool)
        n217 = Not(x=w472) -> (.not. x?=w474:bool)
        n218 = Equal?(x=w482, y=w484) -> (x = y?=w483:bool)
        "NIST Time Failed to Read" <- w483
        n219 = And(x=w475, y=w474) -> (x .and. y?=w473:bool)
        n220 = Select(t=w482, s=w483, f=w484) -> (s? t:f=w485:u64)
        n221 = case shown="True" w473 {
          tunnel: w471 -> [_ w486]
          frame False {
          }
          frame True {
            n222 = To Double Precision Float(number=w486) -> (double precision float=w487:dbl)
            n223 = Multiply(x=2e-08, y=w487) -> (x*y=w489:dbl)
            n224 = To Unsigned Quad Integer(1:w489) -> (0:→"FPGA Timestamp (s)":u64)
          }
        }
        n225 = local read "Write Enable"() -> (w480:bool)
        n226 = Select(t=enum16{"Wait", "Get NIST Time", "Write"}."Write", s=w480, f=enum16{"Wait", "Get NIST Time", "Write"}."Wait") -> (s? t:f=w477:enum16{"Wait", "Get NIST Time", "Write"})
      }
      frame "Write" {
        n227 = local read "Fast Data On"() -> (w492:bool)
        n228 = local read "Slow Control On"() -> (w491:bool)
        n229 = Format Into String(initial string="NIST Time: ", w495) -> (resulting string=w497:string)  [unwired: 2 in, 1 out]
        n230 = case shown="True" w492 {
          tunnel: w495 -> [_ w509]
          tunnel: ["" w507] -> w496
          frame False {
          }
          frame True {
            n231 = local read "FPGA Timestamp (s)"() -> (w510:u64)
            n232 = Subtract(x=w509, y=w510) -> (x-y=w508:u64)
            n233 = Format Into String(initial string="FPGA Time: ", w510) -> (resulting string=w511:string)  [unwired: 2 in, 1 out]
            n234 = Format Into String(initial string="FPGA Drift: ", w508) -> (resulting string=w504:string)  [unwired: 2 in, 1 out]
            n235 = Concatenate Strings(w511, w504) -> (w507:string)
          }
        }
        n236 = case shown="True" w491 {
          tunnel: w495 -> [_ w517]
          tunnel: ["" w513] -> w494
          frame False {
          }
          frame True {
            n237 = local read "Slow time"() -> (w520:u64)
            n238 = Subtract(x=w517, y=w520) -> (x-y=w516:u64)
            n239 = Format Into String(initial string="Slow Drift: ", w516) -> (resulting string=w514:string)  [unwired: 2 in, 1 out]
            n240 = Format Into String(initial string="Slow Data Time: ", w520) -> (resulting string=w515:string)  [unwired: 2 in, 1 out]
            n241 = Concatenate Strings(w515, w514) -> (w513:string)
          }
        }
        n242 = Concatenate Strings(w497, w496, w494, "\r\n") -> (w499:string)
        n243 = Write to Text File(file (use dialog)=w501, text=w499) -> (refnum out=w500:refnum<file>)  [unwired: 2 in, 2 out]
      }
    }
  }
  n244 = case shown="True" w11 {
    tunnel: w13 -> [_ w532]
    tunnel: w7 -> [_ w527]
    tunnel: w6 -> [_ w529]
    tunnel: w1 -> [_ w521]
    frame False {
    }
    frame True {
      n245 = local read "Fast Data On"() -> (w528:bool)
      n246 = case shown="True" w528 {
        tunnel: w527 -> [_ _]
        tunnel: [_ w540] -> w525
        tunnel: w521 -> [_ w541]
        frame False {
        }
        frame True {
          n247 = local read "IP Address of NIST Time Server"() -> (w543:string)
          n248 = call "XML_fast.vi"("Channel Cluster"="Channel Cluster", "DAQ Info Cluster"="DAQ Info Cluster", "Testpulse Cluster"="Testpulse Cluster", "IP Address of NIST Time Server"=w543, "NIST Time"=w541, "General Cluster"="General Cluster") -> ("XML String"=w540:string)  [unwired: 5 in]
          "XML String" <- w540
        }
      }
      n249 = local read "Slow Control On"() -> (w526:bool)
      n250 = case shown="True" w526 {
        tunnel: w525 -> [_ w536]
        tunnel: [_ w537] -> w524
        frame False {
        }
        frame True {
          w538 = "\r\n"
          n251 = local read "Slow Cluster"() -> (w534:T6)
          n252 = call "XML_slow.vi"("Slow Cluster"=w534, "Input String"="") -> ("Output String"=w535:string)
          n253 = Concatenate Strings(w536, w538, w535, w538) -> (w537:string)
        }
      }
      n254 = Close File(refnum=w532) -> ()  [unwired: 1 in, 2 out]
      n255 = Concatenate Strings(w524, "</mod>" ("string")) -> (w522:string)
      n256 = call "UTF8 LV80.vi"("text"=w522) -> ("utf-8 text out"=w531:string)
      n257 = Write to Text File(file (use dialog)=w529, text=w531) -> (refnum out=w530:refnum<file>)  [unwired: 2 in, 2 out]
      n258 = Close File(refnum=w530) -> ()  [unwired: 1 in, 2 out]
    }
  }
